vi "Send_string_to_MCU.vi"() -> (0 "STOP ALL 2":bool)   [LabVIEW 2016]
uses:
  Typedef/MCU_addresses.ctl
  Typedef/Type_of_message_to_MCU.ctl
panel:
  out "error out":errorcluster
  in  "String":string
  in  "Send To MCU":bool
  out "Byte array has been sent":u8[](array[numeric])
  out "Converted Message":string
  in  "Types of Data":T1
  in  "MCU Address to be sent":T2
  in  "EXIT":bool
  in  "STOP ALL":bool
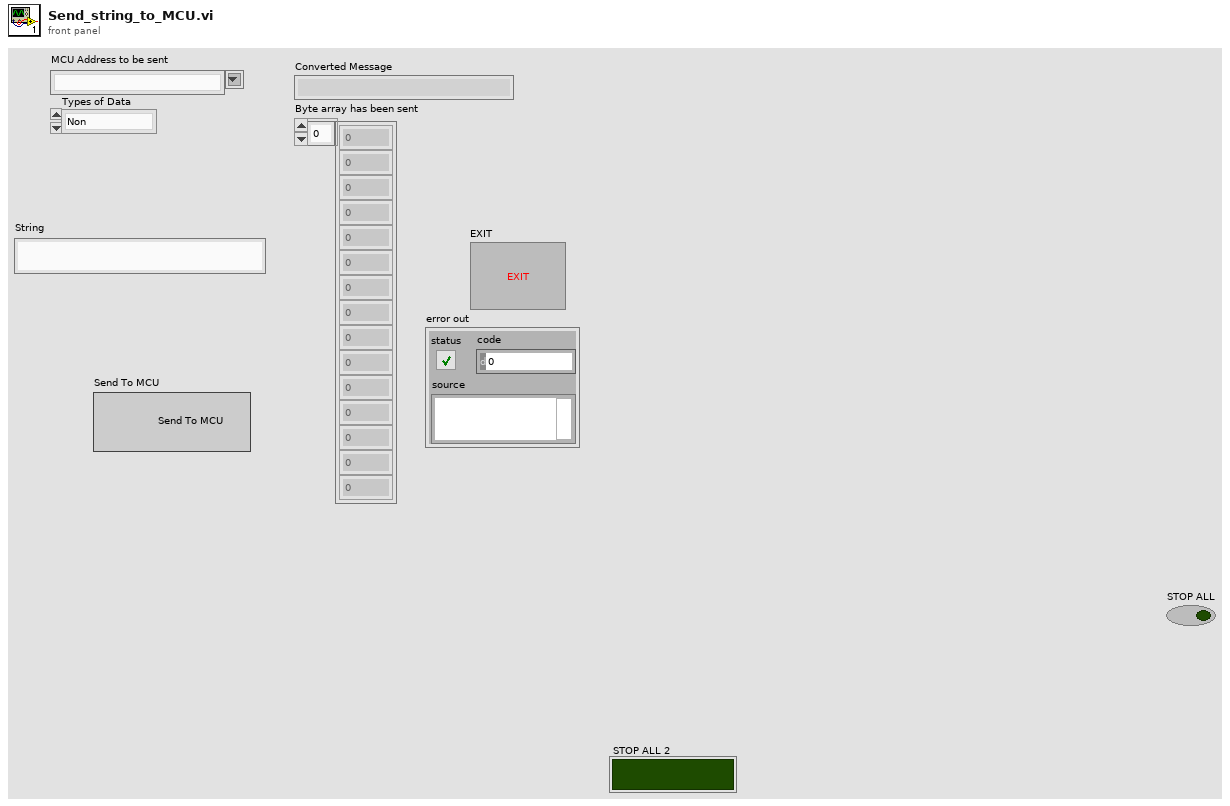
[diagram p1: front panel]
types:
  T1 = typedef "Type_of_message_to_MCU.ctl" = enum16{"Non", "Alarm", "Error", "Time and Date", "Status", "Request"}
  T2 = typedef "MCU_addresses.ctl" = string
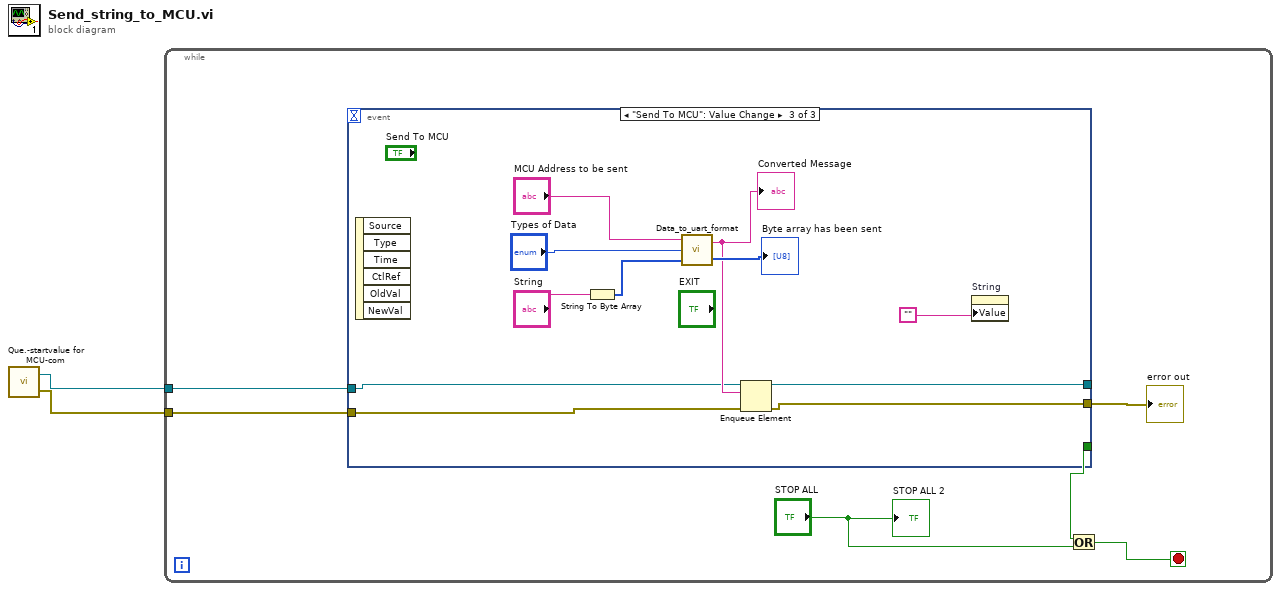
[diagram p0: block diagram]
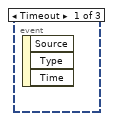
[diagram p2: hidden frame]
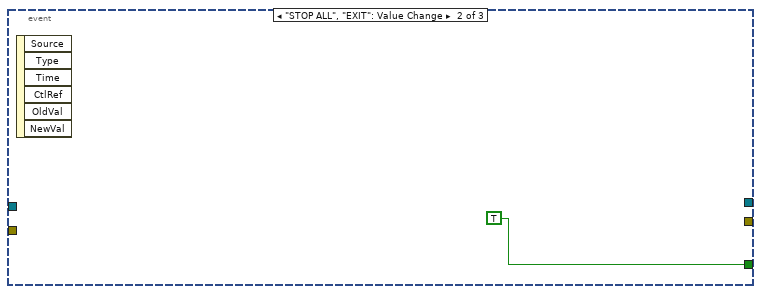
[diagram p3: hidden frame]
diagram:
  n1 = call "Que.-startvalue for MCU-com.vi"() -> ("error out"=w1:errorcluster, "queue out"=w2:refnum<queue>)  [unwired: 2 in]
  n2 = while {
    tunnel: w2 -> [w5]
    tunnel: w1 -> [w4]
    stop <- w6 stop-if-true
    n3 = event shown="[2] \"Send To MCU\": Value Change" {
      selector: _ -> [_ _ _]
      dyn-events: _ -> [_ _ _]
      timeout: _ -> [_ _ _]
      tunnel: [_ TRUE _] -> w7
      tunnel: w5 -> [_ _ w15]
      tunnel: w4 -> [_ _ w14]
      tunnel: [_ _ w11] -> _
      tunnel: [_ _ w10] -> w3
      event Timeout {
        n4 = event-data() -> ()  [unwired: 1 in, 3 out]
      }
      event "STOP ALL", "EXIT": Value Change {
        n5 = event-data() -> ()  [unwired: 1 in, 6 out]
      }
      event "Send To MCU": Value Change {
        n6 = event-data() -> ()  [unwired: 1 in, 6 out]
        n7 = String To Byte Array(string="String") -> (unsigned byte array=w18:u8[])
        n8 = call "Data_to_uart_format.vi"("Payload  Byte to be sent"=w18, "Types of Data"="Types of Data", "MCU Address to be sent"="MCU Address to be sent") -> ("Byte array has been sent"=→"Byte array has been sent":u8[], "Converted Message"=w16:string)
        "Converted Message" <- w16
        n9 = Enqueue Element(queue=w15, element=w16, error in (no error)=w14) -> (queue out=w11:refnum<queue>, error out=w10:errorcluster)  [unwired: 1 in, 1 out]
        n10 = property on="String" class="Str"("Value"="") -> ()  [unwired: 2 in, 2 out]
      }
    }
    "error out" <- w3
    n11 = Or(x=w7, y="STOP ALL") -> (x .or. y?=w6:bool)
    "STOP ALL 2" <- "STOP ALL"
  }
